vi "Destroy UI Events.vi"(11 "Panel in":refnum<class "Panel.lvclass">) -> ()   [LabVIEW 2021, in "Panel.lvclass"]
uses:
  Panel.lvclass
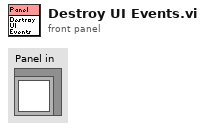
[diagram p1: front panel]
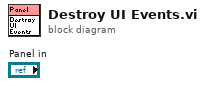
[diagram p0: block diagram]
diagram:
